vi "Open.vi"(1 "error in":errorcluster, 2 "input cluster":T3={"PushSolenoid"=enum."Solenoid 0", "AngleMotor"={"AngleMotor#"=0, "Invert AngleMotor?"=FALSE, "PotScale"=0}, "Wheels"={"LeftWheel#"=0, "Invert LeftWheel?"=FALSE, "RightWheel#"=0, "Invert RightWheel?"=FALSE, "WheelEncoderScale"=0}, "AnglePID"={0.0, 0.0, 0.0}, "WheelPID"={0.0, 0.0, 0.0}, "TopHallDIO"=enum."DIO 9", "BottomHallDIO"=enum."DIO 8"}) -> (0 "error out":errorcluster)   [LabVIEW 2015]
doc: "Opens all refnums used by the firing mechanism."
uses:
  <vilib>/Rock Robotics/WPI/Solenoid/WPI_SolenoidChannel.ctl
  <vilib>/Rock Robotics/SystemInterfaces/DIO/FPGA_DIOChannel.ctl
  <vilib>/Rock Robotics/WPI/CAN/TalonSRX/WPI_CANTalonSRX_APIControlMode.ctl
  <vilib>/Rock Robotics/WPI/SafetyOutput/WPI_SafetyOutputConfigMenu.ctl
  <vilib>/Rock Robotics/WPI/CAN/TalonSRX/WPI_CANTalonSRX_APIFeedbackSelect.ctl
  <vilib>/Rock Robotics/WPI/MotorControl/WPI_MotorControlOpenCANTalonSRX.vi
  <vilib>/Rock Robotics/WPI/Solenoid/WPI_SolenoidOpenSingle.vi
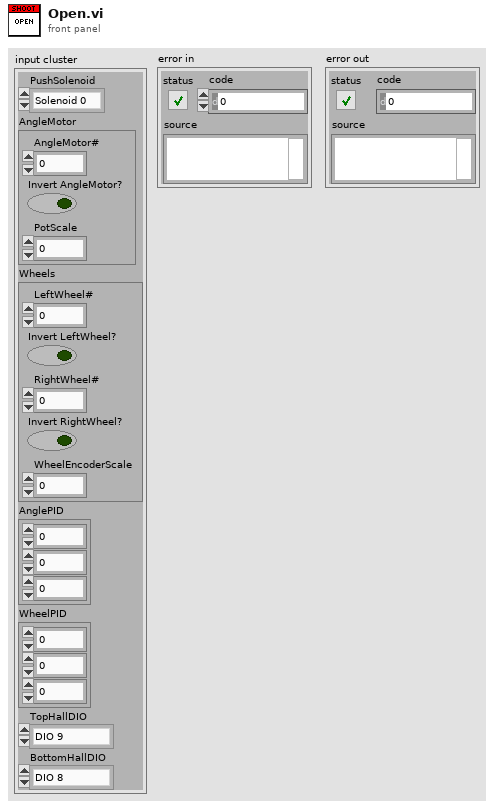
[diagram p1: front panel]
types:
  T1 = typedef "WPI_SolenoidChannel.ctl" = enum8{"Solenoid 0", "Solenoid 1", "Solenoid 2", "Solenoid 3", "Solenoid 4", "Solenoid 5", "Solenoid 6", "Solenoid 7", "Invalid"}
  T2 = typedef "FPGA_DIOChannel.ctl" = enum8{"DIO 0", "DIO 1", "DIO 2", "DIO 3", "DIO 4", "DIO 5", "DIO 6", "DIO 7", "DIO 8", "DIO 9", "DIO MXP 0", "DIO MXP 1", "DIO MXP 2", "DIO MXP 3", "DIO MXP 4", "DIO MXP 5", "DIO MXP 6", "DIO MXP 7", "DIO MXP 8", "DIO MXP 9", "DIO MXP 10", "DIO MXP 11", "DIO MXP 12", "DIO MXP 13", "DIO MXP 14", "DIO MXP 15", "Invalid"}
  T3 = cluster{"PushSolenoid":T1, "AngleMotor":cluster{"AngleMotor#":u8, "Invert AngleMotor?":bool, "PotScale":u32}, "Wheels":cluster{"LeftWheel#":u8, "Invert LeftWheel?":bool, "RightWheel#":u8, "Invert RightWheel?":bool, "WheelEncoderScale":u32}, "AnglePID":cluster{dbl, dbl, dbl}, "WheelPID":cluster{dbl, dbl, dbl}, "TopHallDIO":T2, "BottomHallDIO":T2}
  T4 = typedef "WPI_CANTalonSRX_APIFeedbackSelect.ctl" = enum16{"Digital Quadrature Encoder", "Analog Potentiometer", "Analog Encoder", "Count on Quad-A (Rising-Edge)", "Count on Quad-A (Falling-Edge)", "CTR Magnetic Enc (Absolute)", "CTR Magnetic Enc (Relative)", "Pulse Width"}
  T5 = typedef "WPI_SafetyOutputConfigMenu.ctl" = enum16{"Enable", "Disable"}
  T6 = typedef "WPI_CANTalonSRX_APIControlMode.ctl" = enum8{"Percent VBus", "Speed", "Position", "Slave", "Unchanged / Invalid", "Voltage Compensation", "Current", "Motion Profile"}
  T7 = typedef "WPI_MotorControlDeviceRef.ctl" = cluster{"DeviceStatus":errorcluster, "Type":T8, "PWM":cluster{"PWM Channel":T9, "DeadBand":T10}, "CAN":cluster{"Device Number":u8, "Control Mode":T11, "Semaphore":T12, "Max Vout":dbl, "TalonSRX Control Mode":T6}, "Invert":bool}
  T8 = typedef "WPI_MotorControlType.ctl" = enum16{"PWM", "CAN", "CANTalonSRX"}
  T9 = typedef "FPGA_DIOPWMChannel.ctl" = enum8{"PWM 0", "PWM 1", "PWM 2", "PWM 3", "PWM 4", "PWM 5", "PWM 6", "PWM 7", "PWM 8", "PWM 9", "PWM MXP 0", "PWM MXP 1", "PWM MXP 2", "PWM MXP 3", "PWM MXP 4", "PWM MXP 5", "PWM MXP 6", "PWM MXP 7", "PWM MXP 8", "PWM MXP 9", "Invalid"}
  T10 = typedef "WPI_PWMDeadband.ctl" = cluster{"Name":string, "maxPositivePwm":i32, "minPositivePwm":i32, "centerPwm":i32, "maxNegativePwm":i32, "minNegativePwm":i32, "angularRange":u16}
  T11 = typedef "WPI_CANJaguar_ControlMode.ctl" = enum8{"Percent VBus", "Current", "Speed", "Position", "Voltage"}
  T12 = typedef "Semaphore RefNum" = refnum<k1>
  T13 = typedef "WPI_DigitalInputDevRef.ctl" = cluster{"DevStatus":errorcluster, "DIO Channel":T2}
  T14 = typedef "WPI_SolenoidDevRef.ctl" = cluster{"DevStatus":errorcluster, "Pneumatics Control Module":u8, "Forward Solenoid Channel":T1, "Reverse Solenoid Channel":T1}
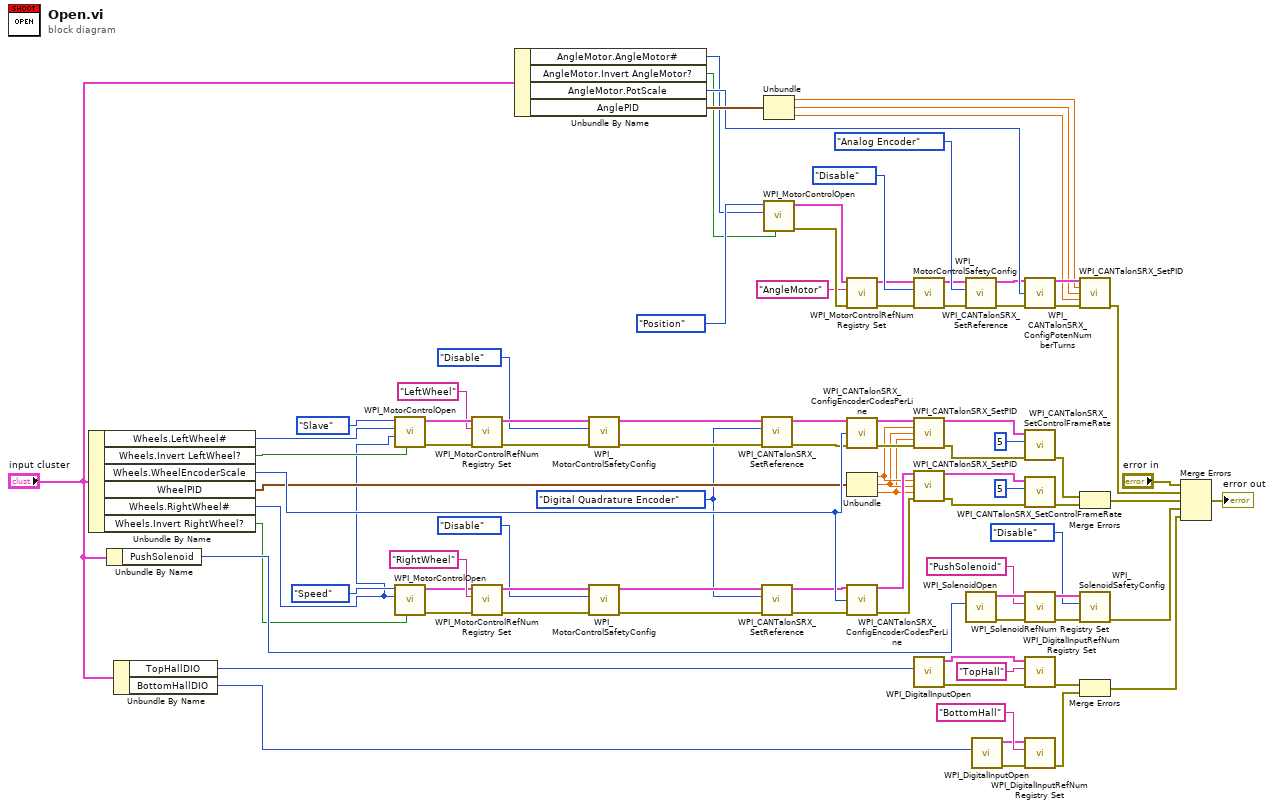
[diagram p0: block diagram]
diagram:
  w10 = WPI_CANTalonSRX_APIFeedbackSelect."Digital Quadrature Encoder" ("Feedback Reference")
  n1 = Unbundle By Name("input cluster") -> ("Wheels.LeftWheel#"=w71:u8, "Wheels.Invert LeftWheel?"=w70:bool, "Wheels.WheelEncoderScale"=w43:u32, "WheelPID"=w42:cluster{dbl, dbl, dbl}, "Wheels.RightWheel#"=w1:u8, "Wheels.Invert RightWheel?"=w39:bool)
  n2 = Unbundle By Name("input cluster") -> ("PushSolenoid"=w66:T1)
  n3 = Unbundle By Name("input cluster") -> ("TopHallDIO"=w27:T2, "BottomHallDIO"=w26:T2)
  n4 = call-poly <vilib>:"WPI_MotorControlOpen.vi"("Invert"=w70, "Master Device Number"=w1, "Device Number"=w71, "Control Mode"=WPI_CANTalonSRX_APIControlMode."Slave") -> ("error out"=w87:errorcluster, "MotorControlDeviceRef"=w86:T7)  [unwired: 6 in]
  n5 = call-poly <vilib>:"WPI_MotorControlOpen.vi"("Invert"=w39, "Device Number"=w1, "Control Mode"=WPI_CANTalonSRX_APIControlMode."Speed") -> ("error out"=w76:errorcluster, "MotorControlDeviceRef"=w78:T7)  [unwired: 7 in]
  n6 = call <vilib>:"WPI_MotorControlRefNum Registry Set.vi"("error in (no error)"=w87, "refnum name"="LeftWheel", "MotorControlDevRef"=w86) -> ("error out"=w73:errorcluster, "MotorControlDevRef"=w72:T7)  [unwired: 7 in]
  n7 = call <vilib>:"WPI_MotorControlRefNum Registry Set.vi"("error in (no error)"=w76, "refnum name"="RightWheel", "MotorControlDevRef"=w78) -> ("error out"=w75:errorcluster, "MotorControlDevRef"=w74:T7)  [unwired: 7 in]
  n8 = Unbundle By Name("input cluster") -> ("AngleMotor.AngleMotor#"=w40:u8, "AngleMotor.Invert AngleMotor?"=w41:bool, "AngleMotor.PotScale"=w45:u32, "AnglePID"=w48:cluster{dbl, dbl, dbl})
  n9 = call <vilib>:"WPI_MotorControlSafetyConfig.vi"("error in (no error)"=w73, "mode"=WPI_SafetyOutputConfigMenu."Disable", "MotorControlDevRef"=w72) -> ("error out"=w17:errorcluster, "MotorControlDevRef"=w18:T7)  [unwired: 7 in]
  n10 = call <vilib>:"WPI_MotorControlSafetyConfig.vi"("error in (no error)"=w75, "mode"=WPI_SafetyOutputConfigMenu."Disable", "MotorControlDevRef"=w74) -> ("error out"=w13:errorcluster, "MotorControlDevRef"=w14:T7)  [unwired: 7 in]
  n11 = call <vilib>:"WPI_CANTalonSRX_SetReference.vi"("error in (no error)"=w17, "Feedback Reference"=w10, "CAN Talon SRX Ref"=w18) -> ("error out"=w15:errorcluster, "CAN Talon SRX Ref"=w16:T7)  [unwired: 7 in]
  n12 = call <vilib>:"WPI_CANTalonSRX_SetReference.vi"("error in (no error)"=w13, "Feedback Reference"=w10, "CAN Talon SRX Ref"=w14) -> ("error out"=w11:errorcluster, "CAN Talon SRX Ref"=w12:T7)  [unwired: 7 in]
  n13 = Unbundle(w48) -> (w54:dbl, w53:dbl, w52:dbl)
  n14 = call-poly <vilib>:"WPI_MotorControlOpen.vi"("Invert"=w41, "Device Number"=w40, "Control Mode"=WPI_CANTalonSRX_APIControlMode."Position") -> ("error out"=w89:errorcluster, "MotorControlDeviceRef"=w88:T7)  [unwired: 7 in]
  n15 = call <vilib>:"WPI_MotorControlRefNum Registry Set.vi"("error in (no error)"=w89, "refnum name"="AngleMotor", "MotorControlDevRef"=w88) -> ("error out"=w62:errorcluster, "MotorControlDevRef"=w22:T7)  [unwired: 7 in]
  n16 = call <vilib>:"WPI_CANTalonSRX_ConfigEncoderCodesPerLine.vi"("CAN Talon SRX Ref"=w16, "Number Encoder Lines\n(Counts Per Rotation)"=w43, "error in (no error)"=w15) -> ("CAN Talon SRX Ref"=w59:T7, "error out"=w58:errorcluster)  [unwired: 11 in]
  n17 = Unbundle(w42) -> (w51:dbl, w50:dbl, w49:dbl)
  n18 = call <vilib>:"WPI_CANTalonSRX_ConfigEncoderCodesPerLine.vi"("CAN Talon SRX Ref"=w12, "Number Encoder Lines\n(Counts Per Rotation)"=w43, "error in (no error)"=w11) -> ("CAN Talon SRX Ref"=w56:T7, "error out"=w55:errorcluster)  [unwired: 11 in]
  n19 = call <vilib>:"WPI_MotorControlSafetyConfig.vi"("error in (no error)"=w62, "mode"=WPI_SafetyOutputConfigMenu."Disable", "MotorControlDevRef"=w22) -> ("error out"=w20:errorcluster, "MotorControlDevRef"=w23:T7)  [unwired: 7 in]
  n20 = call <vilib>:"WPI_CANTalonSRX_SetPID.vi"("CAN Talon SRX Ref"=w59, "P"=w51, "I"=w50, "D"=w49, "error in (no error)"=w58) -> ("CAN Talon SRX Ref"=w7:T7, "error out"=w6:errorcluster)  [unwired: 9 in]
  n21 = call <vilib>:"WPI_CANTalonSRX_SetPID.vi"("CAN Talon SRX Ref"=w56, "P"=w51, "I"=w50, "D"=w49, "error in (no error)"=w55) -> ("CAN Talon SRX Ref"=w4:T7, "error out"=w5:errorcluster)  [unwired: 9 in]
  n22 = call <vilib>:"WPI_DigitalInputOpen.vi"("DIO Channel"=w27) -> ("error out"=w34:errorcluster, "DigitalInputDevRef"=w36:T13)  [unwired: 9 in]
  n23 = call <vilib>:"WPI_CANTalonSRX_SetReference.vi"("error in (no error)"=w20, "Feedback Reference"=WPI_CANTalonSRX_APIFeedbackSelect."Analog Encoder", "CAN Talon SRX Ref"=w23) -> ("error out"=w19:errorcluster, "CAN Talon SRX Ref"=w21:T7)  [unwired: 7 in]
  n24 = call-poly <vilib>:"WPI_SolenoidOpen.vi"("Solenoid Channel"=w66) -> ("error out"=w68:errorcluster, "SolenoidDevRef"=w69:T14)  [unwired: 9 in]
  n25 = call <vilib>:"WPI_DigitalInputOpen.vi"("DIO Channel"=w26) -> ("error out"=w33:errorcluster, "DigitalInputDevRef"=w31:T13)  [unwired: 9 in]
  n26 = call <vilib>:"WPI_CANTalonSRX_ConfigPotenNumberTurns.vi"("CAN Talon SRX Ref"=w21, "Number Potentiometer Turns"=w45, "error in (no error)"=w19) -> ("CAN Talon SRX Ref"=w61:T7, "error out"=w60:errorcluster)  [unwired: 11 in]
  n27 = call <vilib>:"WPI_CANTalonSRX_SetControlFrameRate.vi"("error in (no error)"=w6, "Control Frame Rate (ms)"=u8 5, "CAN Talon SRX Ref"=w7) -> ("error out"=w2:errorcluster)  [unwired: 7 in, 1 out]
  n28 = call <vilib>:"WPI_CANTalonSRX_SetControlFrameRate.vi"("error in (no error)"=w5, "Control Frame Rate (ms)"=u8 5, "CAN Talon SRX Ref"=w4) -> ("error out"=w3:errorcluster)  [unwired: 7 in, 1 out]
  n29 = call <vilib>:"WPI_SolenoidRefNum Registry Set.vi"("error in (no error)"=w68, "refnum name"="PushSolenoid", "SolenoidDevRef"=w69) -> ("error out"=w65:errorcluster, "SolenoidDevRef"=w63:T14)  [unwired: 7 in]
  n30 = call <vilib>:"WPI_DigitalInputRefNum Registry Set.vi"("error in (no error)"=w34, "refnum name"="TopHall", "DigitalInputDevRef"=w36) -> ("error out"=w30:errorcluster)  [unwired: 7 in, 1 out]
  n31 = call <vilib>:"WPI_DigitalInputRefNum Registry Set.vi"("error in (no error)"=w33, "refnum name"="BottomHall", "DigitalInputDevRef"=w31) -> ("error out"=w29:errorcluster)  [unwired: 7 in, 1 out]
  n32 = call <vilib>:"WPI_CANTalonSRX_SetPID.vi"("CAN Talon SRX Ref"=w61, "P"=w54, "I"=w53, "D"=w52, "error in (no error)"=w60) -> ("error out"=w57:errorcluster)  [unwired: 9 in, 1 out]
  n33 = Merge Errors(w2, w3) -> (w37:errorcluster)
  n34 = call <vilib>:"WPI_SolenoidSafetyConfig.vi"("error in (no error)"=w65, "mode"=WPI_SafetyOutputConfigMenu."Disable", "SolenoidDevRef"=w63) -> ("error out"=w38:errorcluster)  [unwired: 7 in, 1 out]
  n35 = Merge Errors(w30, w29) -> (w28:errorcluster)
  n36 = Merge Errors("error in", w57, w37, w38, w28) -> (→"error out":errorcluster)
